vi "arduino Motor Control Driver Generate Command String.vi"(8 "error in (no error)":errorcluster, 10 "Command":T1={"Direction"=TRUE, "NUMBER OF  STEPS"=13000, "SPEED STEPS/SEC"=1000, "ACC/DECEL STEPS/SEC^2"=1000, "EN/DIS?"=TRUE} {"ACC/DECEL STEPS/SEC^2" max=4000; "SPEED STEPS/SEC" min=20 max=4000 step=10}, 11 "MOTOR NUMBER":u8 max=3 step=1) -> (0 "error out":errorcluster, 3 "Cmd String":string)   [LabVIEW 2024]
uses:
  arduino Motor Control cluster Command.ctl
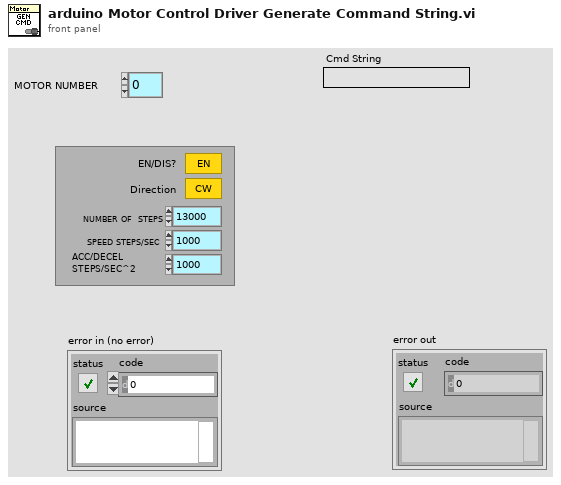
[diagram p1: front panel]
types:
  T1 = typedef "arduino Motor Control cluster Command.ctl" = cluster{"Direction":bool, "NUMBER OF  STEPS":u32, "SPEED STEPS/SEC":u16, "ACC/DECEL STEPS/SEC^2":u16, "EN/DIS?":bool}
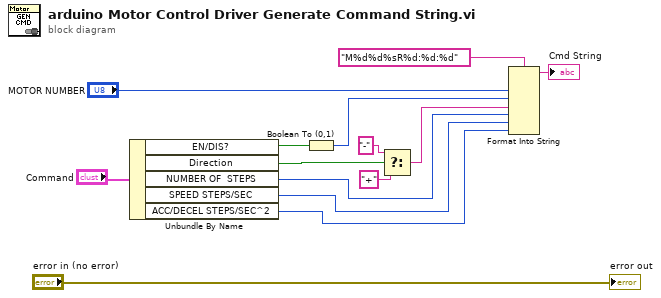
[diagram p0: block diagram]
diagram:
  n1 = Unbundle By Name("Command") -> ("EN/DIS?"=w11:bool, "Direction"=w9:bool, "NUMBER OF  STEPS"=w5:u32, "SPEED STEPS/SEC"=w4:u16, "ACC/DECEL STEPS/SEC^2"=w3:u16)
  n2 = Boolean To (0,1)(Boolean=w11) -> (0, 1=w10:i16)
  n3 = Select(t="-", s=w9, f="+") -> (s? t:f=w6:string)
  n4 = Format Into String(format string="M%d%d%sR%d:%d:%d", "MOTOR NUMBER", w10, w6, w5, w4, w3) -> (resulting string=→"Cmd String":string)  [unwired: 2 in, 1 out]
  "error out" <- "error in (no error)"
